vi "epoch access point to epoch millisecond.vi"(11 "sync_value":cluster{}) -> (3 "function return":u64)   [LabVIEW 2019, in "apdm.lvlib"]
doc: "APDM_EXPORT uint64_t apdm_epoch_access_point_to_epoch_millisecond(const uint64_t sync_value);"
uses:
  apdm.lvlib
  Lee Lab/CP FES Walking 2018/Code/Working/LabVIEW/apdm.dll
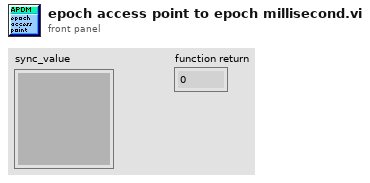
[diagram p1: front panel]
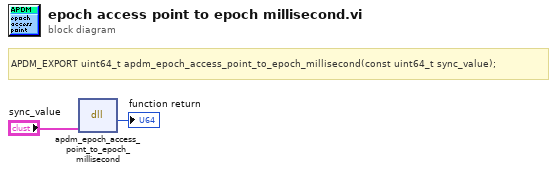
[diagram p0: block diagram]
diagram:
  # "APDM_EXPORT uint64_t apdm_epoch_access_point_to_epoch_millisecond(const uint64_t sync_value);"
  n1 = dll-call lib="C:/Users/jfalesi/Dropbox/Lee Lab/CP FES Walking 2018/Code/Working/LabVIEW/apdm.*" fn="apdm_epoch_access_point_to_epoch_millisecond"("sync_value"="sync_value") -> (→"function return":u64)  [unwired: 4 in, 2 out]
